vi "Write Value.vi"(8 "error in (no error)":errorcluster caption="entrée d'erreur (pas d'erreur)", 10 "Data":string, 11 "DAQmxTaskDOutput en entrée":refnum<class "DAQmxTaskDOutput.lvclass">) -> (0 "error out":errorcluster caption="sortie d'erreur", 3 "DAQmxTaskDOutput en sortie":refnum<class "DAQmxTaskDOutput.lvclass">)   [LabVIEW 2015, in "DAQmxTaskDOutput.lvclass"]
uses:
  DAQmxTaskDOutput.lvclass
  DAQmxTask.lvclass/DAQmxTask.ctl
  <vilib>/DAQmx/write.llb/DAQmx Write (Digital Bool 1Line 1Point).vi
  <vilib>/DAQmx/miscellaneous.llb/DAQmx Fill In Error Info.vi
  DAQmxTask.lvclass
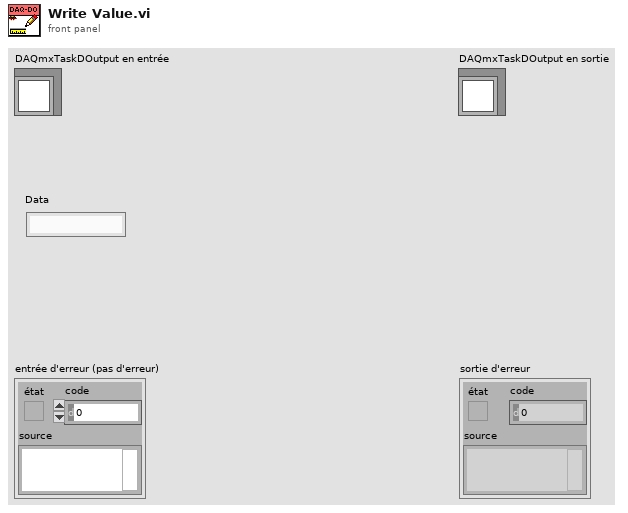
[diagram p1: front panel]
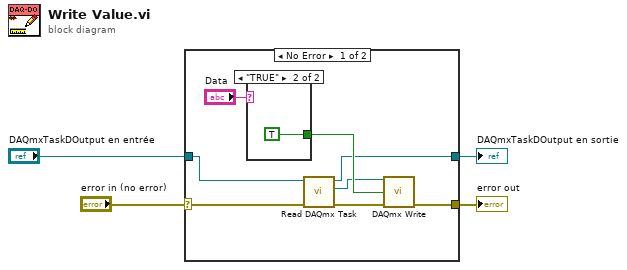
[diagram p0: block diagram]
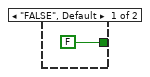
[diagram p2: hidden frame]
diagram:
  n1 = case shown="No Error" "error in (no error)" {
    selector: "error in (no error)" -> [w10 w16]
    tunnel: [w7 w16] -> w3
    tunnel: [w5 w15] -> w2
    tunnel: "DAQmxTaskDOutput en entrée" -> [w11 w15]
    frame No Error {
      n2 = case shown="\"TRUE\"" "Data" {
        tunnel: [FALSE TRUE] -> w12
        frame "FALSE", Default {
        }
        frame "TRUE" {
        }
      }
      n3 = call "Read DAQmx Task.vi"("error in (no error)"=w10, "DAQmxTask in"=w11) -> ("error out"=w8:errorcluster, "DAQmx Task Name"=w9:refnum<k21>, "DAQmxTask out"=w5:refnum<class "DAQmxTaskDOutput.lvclass">)  [unwired: 7 in]
      n4 = call-poly <vilib>:"DAQmx Write.vi"("task/channels in"=w9, "data"=w12, "error in"=w8) -> ("error out"=w7:errorcluster)  [unwired: 10 in, 2 out]
    }
    frame Error {
    }
  }
  "error out" <- w3
  "DAQmxTaskDOutput en sortie" <- w2
